vi "Write MSG.vi"(8 "error in (no error)":errorcluster, 10 "Actor Framework:Message":refnum<class "Message.lvclass">, 11 "Send MSG STEP in":refnum<class "Send MSG STEP.lvclass">) -> (0 "error out":errorcluster, 3 "Send MSG STEP out":refnum<class "Send MSG STEP.lvclass">)   [LabVIEW 2014, in "Send MSG STEP.lvlib" / "Send MSG STEP.lvclass"]
uses:
  Send MSG STEP.lvclass
  <vilib>/ActorFramework/Message/Message.lvclass
  Send MSG STEP.lvclass/Send MSG STEP.ctl
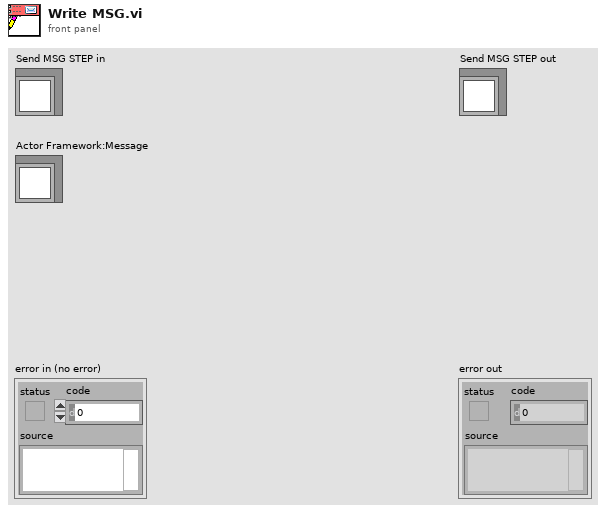
[diagram p1: front panel]
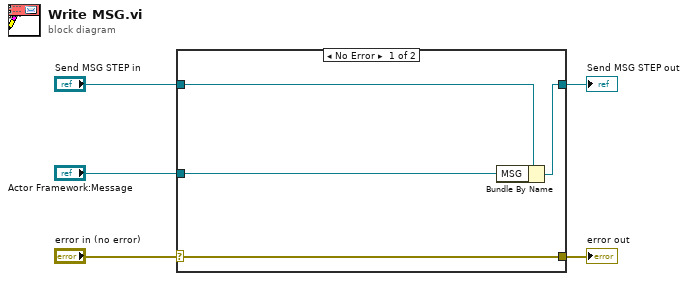
[diagram p0: block diagram]
diagram:
  n1 = case shown="No Error" "error in (no error)" {
    selector: "error in (no error)" -> [w9 w10]
    tunnel: [w9 w10] -> w4
    tunnel: [w7 w11] -> w2
    tunnel: "Send MSG STEP in" -> [w8 w11]
    tunnel: "Actor Framework:Message" -> [w6 _]
    frame No Error {
      n2 = Bundle By Name(cluster=w8, "MSG"=w6) -> (w7:refnum<class "Send MSG STEP.lvclass">)
    }
    frame Error {
    }
  }
  "error out" <- w4
  "Send MSG STEP out" <- w2
